vi "Load XML File.vi"(0 "path to XML document":path, 1 "preserve whitespace (True)":bool=TRUE, 2 "validate on load (Auto)":i32(ring)=2 items=["Never", "Always", "Auto"], 5 "process namespaces (False)":bool, 7 "process schema (False)":bool, 9 "load external DTD (True)":bool=TRUE, 11 "error in (no error)":errorcluster, 12 "schema full checking (False)":bool) -> (4 "DOM document out":refnum<k20>, 6 "parse errors":string, 15 "error out":errorcluster)   [LabVIEW 2017, in "NI_XML.lvlib"]
doc: "Opens an XML file and allows you to configure the XML parser to validate the file against a schema or Document Type Definition (DTD).\n\nNational Instruments recommends that you use the Close VI to close all the references after using the XML parser classes."
uses:
  <vilib>/xml/NI_XML.lvlib
  <resource>/objmgr/DOMUserDefRef.rc
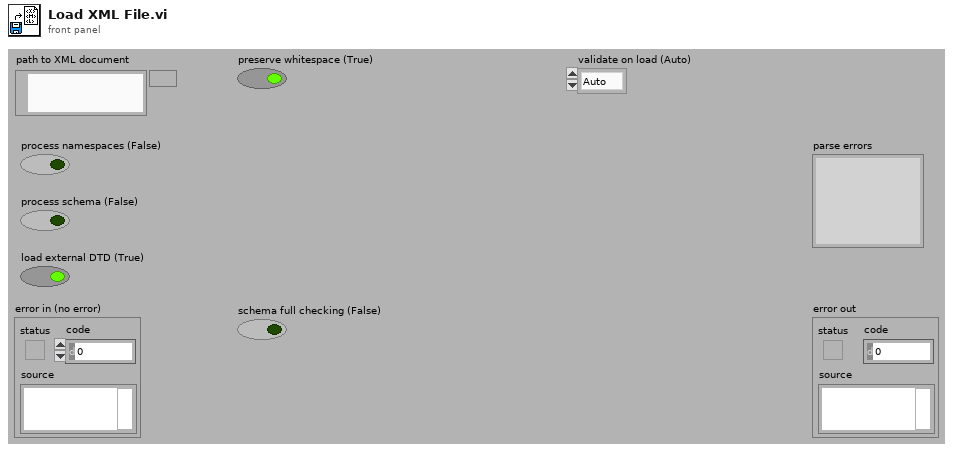
[diagram p1: front panel]
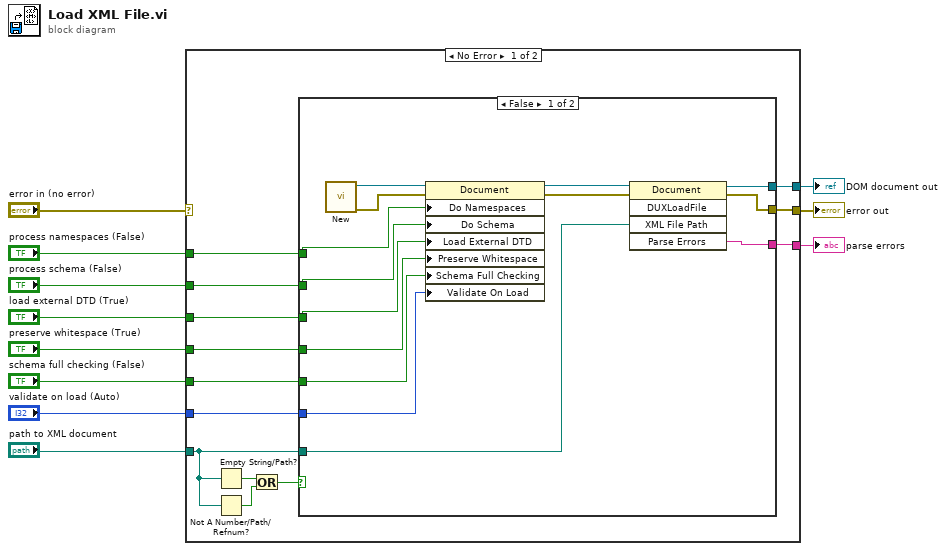
[diagram p0: block diagram]
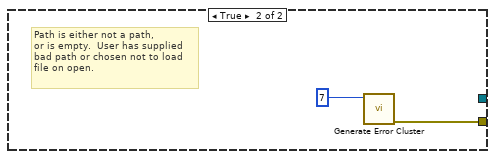
[diagram p2: hidden frame]
diagram:
  n1 = case shown="No Error" "error in (no error)" {
    selector: "error in (no error)" -> [_ w41]
    tunnel: [w23 _] -> w11
    tunnel: [w22 w41] -> w10
    tunnel: "path to XML document" -> [w19 _]
    tunnel: [w24 _] -> w7
    tunnel: "validate on load (Auto)" -> [w17 _]
    tunnel: "schema full checking (False)" -> [w16 _]
    tunnel: "preserve whitespace (True)" -> [w15 _]
    tunnel: "load external DTD (True)" -> [w14 _]
    tunnel: "process schema (False)" -> [w13 _]
    tunnel: "process namespaces (False)" -> [w12 _]
    frame No Error {
      n2 = Empty String/Path?(string/path=w19) -> (empty?=w21:bool)
      n3 = Not A Number/Path/Refnum?(number/path/refnum=w19) -> (NaN/Path/Refnum?=w20:bool)
      n4 = Or(x=w21, y=w20) -> (x .or. y?=w18:bool)
      n5 = case shown="False" w18 {
        tunnel: [w38 _] -> w24
        tunnel: [w33 _] -> w23
        tunnel: [w32 w39] -> w22
        tunnel: w19 -> [w31 _]
        tunnel: w17 -> [w30 _]
        tunnel: w16 -> [w29 _]
        tunnel: w15 -> [w28 _]
        tunnel: w14 -> [w27 _]
        tunnel: w13 -> [w26 _]
        tunnel: w12 -> [w25 _]
        frame False {
          n6 = call <vilib>:"New.vi"() -> ("error out"=w36:errorcluster, "DOM document out"=w37:refnum<k20>)  [unwired: 1 in, 7 out]
          n7 = property class="Document"(reference=w37, error in=w36, "Do Namespaces"=w25, "Do Schema"=w26, "Load External DTD"=w27, "Preserve Whitespace"=w28, "Schema Full Checking"=w29, "Validate On Load"=w30) -> (reference out=w35:refnum<k20>, error out=w34:errorcluster)
          n8 = invoke class="Document" method="DUXLoadFile"(reference=w35, error in=w34, "XML File Path"=w31) -> (reference out=w33:refnum<k20>, error out=w32:errorcluster, "Parse Errors"=w38:string)  [unwired: 2 in, 2 out]
        }
        frame True {
          # "Path is either not a path,\nor is empty.  User has supplied\nbad path or chosen not to load\nfile on open."
          n9 = call <vilib>:"Generate Error Cluster.vi"("Code"=7) -> ("error out"=w39:errorcluster)  [unwired: 2 in, 8 out]
        }
      }
    }
    frame Error {
    }
  }
  "DOM document out" <- w11
  "error out" <- w10
  "parse errors" <- w7
